vi "initialize.vi"(8 "error in (no error)":errorcluster, 11 "lv-builder-l3 in":refnum<class "lv-builder-l3.lvclass">) -> (0 "error out":errorcluster, 3 "lv-builder-l3 out":refnum<class "lv-builder-l3.lvclass">)   [LabVIEW 2015, in "lv-builder-l3.lvlib" / "lv-builder-l3.lvclass"]
uses:
  lv-builder-l3.lvclass
  <userlib>/antonio-alexander/lv-bin/public/api/v1/advanced/add_data_path_single.vi
  lv-builder-l3.lvlib
  <userlib>/antonio-alexander/lv-bin-git/public/api/v1/v1.lvlib
  <userlib>/antonio-alexander/lv-bin-git/lv-bin-git.lvlib
  <userlib>/antonio-alexander/lv-bin-7zip/lv-bin-7zip.lvlib
  <userlib>/antonio-alexander/lv-bin/public/api/v1/v1.lvlib
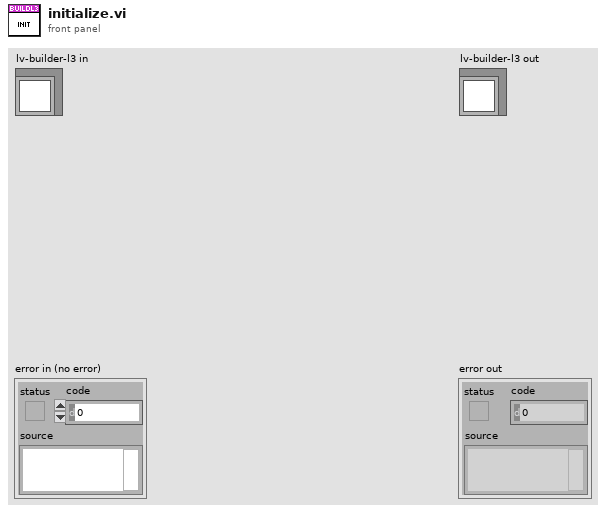
[diagram p1: front panel]
types:
  T1 = typedef "lv-builder-l3.lvlib/configuration.ctl" = cluster{"project_file":string, "l3_archive_file_path":string}
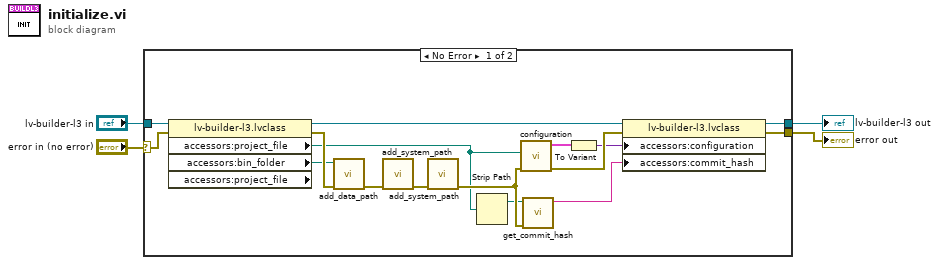
[diagram p0: block diagram]
diagram:
  n1 = case shown="No Error" "error in (no error)" {
    selector: "error in (no error)" -> [w17 w22]
    tunnel: "lv-builder-l3 in" -> [w16 w21]
    tunnel: [w11 w21] -> w2
    tunnel: [w10 w22] -> w1
    frame No Error {
      n2 = property class="lv-builder-l3.lvclass" props=["accessors:project_file", "accessors:bin_folder", "accessors:project_file"](reference=w16, error in=w17) -> (reference out=w12:refnum<class "lv-builder-l3.lvclass">, error out=w18:errorcluster, "accessors:project_file"=w6:path, "accessors:bin_folder"=w5:path)  [unwired: 1 out]
      n3 = call-poly <userlib>:"add_data_path.vi"("error in (no error)"=w18, "path_to_add"=w5) -> ("error out"=w15:errorcluster)  [unwired: 9 in]
      n4 = call <userlib>:"add_system_path.vi"("error in (no error)"=w15) -> ("error out"=w14:errorcluster)  [unwired: 10 in]
      n5 = call <userlib>:"add_system_path.vi"("error in (no error)"=w14) -> ("error out"=w19:errorcluster)  [unwired: 10 in]
      n6 = Strip Path(path=w6) -> (stripped path=w9:path)  [unwired: 1 out]
      n7 = call "configuration.vi"("error in (no error)"=w19, "project_file"=w6) -> ("error out"=w20:errorcluster, "config out"=w8:T1)  [unwired: 8 in]
      n8 = call <userlib>:"get_commit_hash.vi"("error in (no error)"=w19, "path"=w9) -> ("commit_hash"=w7:string)  [unwired: 8 in, 1 out]
      n9 = To Variant(anything=w8) -> (Variant=w13:variant)
      n10 = property class="lv-builder-l3.lvclass"(reference=w12, error in=w20, "accessors:configuration"=w13, "accessors:commit_hash"=w7) -> (reference out=w11:refnum<class "lv-builder-l3.lvclass">, error out=w10:errorcluster)
    }
    frame Error {
    }
  }
  "error out" <- w1
  "lv-builder-l3 out" <- w2
